vi "Logging Delete Tree Item.vi"(2 "Name":string, 3 "TreeRef":refnum<vi>) -> (1 "TreeRef":refnum<vi>)   [LabVIEW 2012, in "femtoRoboLib.lvlib"]
uses:
  femtoRoboLib.lvlib
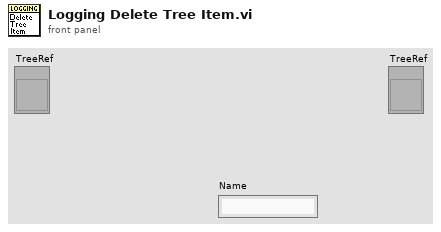
[diagram p1: front panel]
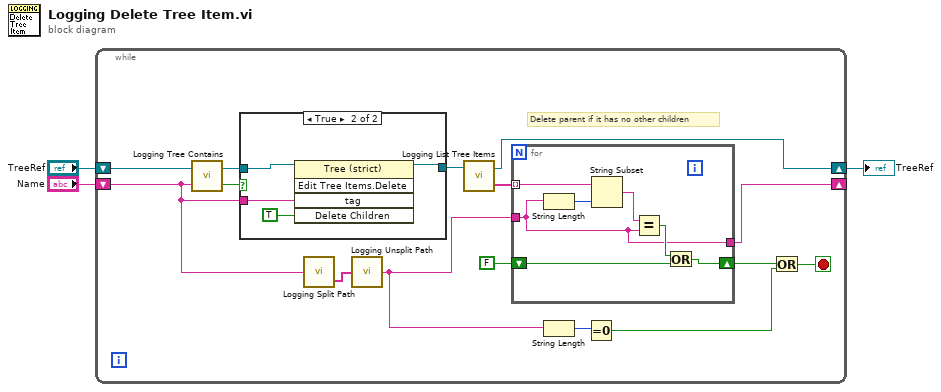
[diagram p0: block diagram]
diagram:
  n1 = while {
    shift-right: [w4] -> _
    shift-left: "Name" -> [w15]
    shift-right: [w6] -> w1
    shift-left: "TreeRef" -> [w16]
    stop <- w8 stop-if-true
    # "Delete parent if it has no other children"
    n2 = call "Logging Tree Contains.vi"("Name"=w15, "TreeRef"=w16) -> ("Contained"=w18:bool, "TreeRef"=w17:refnum<vi>)
    n3 = case shown="True" w18 {
      tunnel: w17 -> [w26 w30]
      tunnel: [w26 w27] -> w13
      tunnel: w15 -> [_ w29]
      frame False {
      }
      frame True {
        n4 = invoke class="Tree (strict)" method="Edit Tree Items.Delete"(reference=w30, "tag"=w29, "Delete Children"=TRUE ("Delete Children?")) -> (reference out=w27:refnum<vi>)  [unwired: 2 in, 4 out]
      }
    }
    n5 = call "Logging Split Path.vi"("Path In"=w15) -> ("Split Path"=w14:string[])  [unwired: 1 out]
    n6 = call "Logging Unsplit Path.vi"("Split Path"=w14) -> ("Path"=w10:string)
    n7 = call "Logging List Tree Items.vi"("TreeRef"=w13) -> ("Items"=w12:string[], "TreeRef"=w6:refnum<vi>)  [unwired: 1 in]
    n8 = for {
      tunnel: w12 -> [w25] mode=indexing
      tunnel: w10 -> [w19]
      shift-right: [w22] -> w5
      shift-left: FALSE -> [w21]
      tunnel: [w19] -> w4
      n9 = String Length(string=w19) -> (length=w24:i32)
      n10 = String Subset(string=w25, length (rest)=w24) -> (substring=w20:string)  [unwired: 1 in]
      n11 = Equal?(x=w20, y=w19) -> (x = y?=w23:bool)
      n12 = Or(x=w23, y=w21) -> (x .or. y?=w22:bool)
    }
    n13 = String Length(string=w10) -> (length=w9:i32)
    n14 = Equal To 0?(x=w9) -> (x = 0?=w7:bool)
    n15 = Or(x=w5, y=w7) -> (x .or. y?=w8:bool)
  }
  "TreeRef" <- w1
